vi "store_documents.vi"(0 "destination_vectorstore in":refnum<class "destination_vectorstore.lvclass">, 5 "documents":refnum<class "data_document.lvclass">[](array[class]), 11 "error in (no error)":errorcluster) -> (4 "destination_vectorstore out":refnum<class "destination_vectorstore.lvclass">, 15 "error out":errorcluster)   [LabVIEW 2020, in "destination_vectorstore.lvclass"]
uses:
  destination_vectorstore.lvclass
  data/data_document/data_document.lvclass
  destination_vectorstore.lvclass/destination_vectorstore.ctl
  vectorstore/abstract_vector_base/vector.ctl
  vectorstore/abstract_vector_base/abstract_vector_base.lvclass
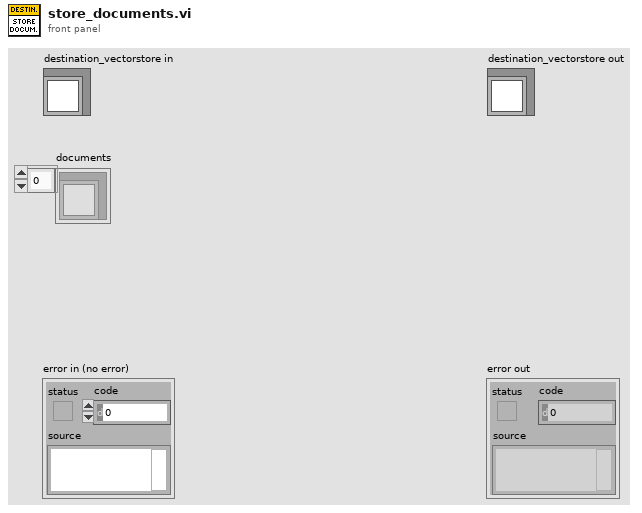
[diagram p1: front panel]
types:
  T1 = typedef "abstract_vector_base.lvclass/vector.ctl" = cluster{"id":string, "vector":dbl[], "text":string, "metadata":cluster{"key":string, "value":string}[]}
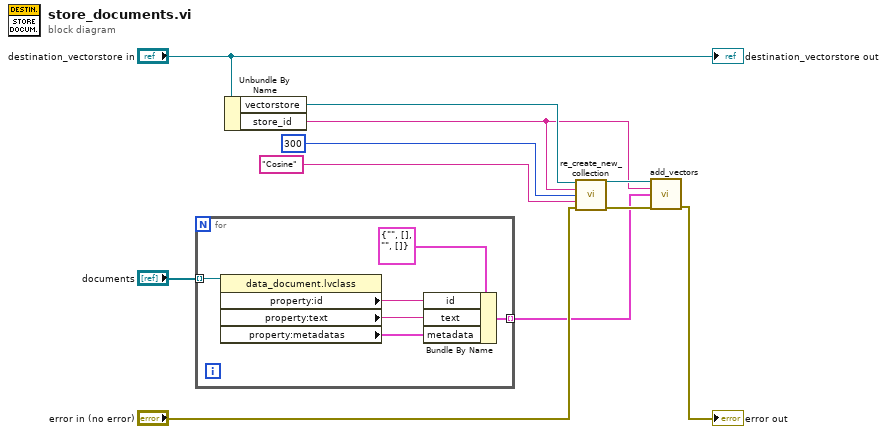
[diagram p0: block diagram]
diagram:
  n1 = for {
    tunnel: "documents" -> [w17] mode=indexing
    tunnel: [w12] -> w1 mode=indexing
    n2 = property class="data_document.lvclass"(reference=w17) -> ("property:id"=w15:string, "property:text"=w14:string, "property:metadatas"=w13:cluster{"key":string, "value":string}[])  [unwired: 1 in, 2 out]
    n3 = Bundle By Name(cluster=T1 {"id"="", "vector"=[], "text"="", "metadata"=[]} ("vector"), "id"=w15, "text"=w14, "metadata"=w13) -> (w12:T1)
  }
  n4 = Unbundle By Name("destination_vectorstore in") -> ("vectorstore"=w7:refnum<class "abstract_vector_base.lvclass">, "store_id"=w6:string)
  n5 = call-dynamic "re_create_new_collection.vi"("abstract_vector_base in"=w7, "collection_name"=w6, "vector_size"=u32 300, "distance"="Cosine", "error in (no error)"="error in (no error)") -> ("abstract_vector_base out"=w9:refnum<class "abstract_vector_base.lvclass">, "error out"=w8:errorcluster)  [unwired: 9 in]
  n6 = call-dynamic "add_vectors.vi"("abstract_vector_base in"=w9, "colection_name"=w6, "vectors"=w1, "error in (no error)"=w8) -> ("error out"=→"error out":errorcluster)  [unwired: 10 in, 1 out]
  "destination_vectorstore out" <- "destination_vectorstore in"
